vi "Publish Data.vi"(7 "Message Priority (Normal)":T1, 9 "Data":refnum<class "Data.lvclass">, 10 "Actor in":refnum<class "Actor.lvclass">, 11 "Response Msg":refnum<class "Response Msg.lvclass">) -> (0 "error out":errorcluster, 2 "Actor out":refnum<class "Actor.lvclass">)   [LabVIEW 2020, in "Publisher.lvlib" / "Response Msg.lvclass"]
doc: "This Vi handles the publishing of the Data from the Response Msg.\n\nThe default implementation publishes Data if it is non-empty."
uses:
  Response Msg.lvclass
  PPL/HDH.Data.Generic.lvlibp/Data.lvclass
  PPL/HDH.Actor Framework.Core.Actor.lvlibp/1abvi3w/vi.lib/ActorFramework/Actor/Actor.lvclass
  PPL/HDH.Actor Framework.Core.Actor.lvlibp/1abvi3w/vi.lib/ActorFramework/Message Enqueuer/Message Priority.ctl
  Data Msg/Data Msg.lvclass/Data Msg.ctl
  Publisher Messages/Publish Msg/Publish Msg.lvclass/Publish Msg.ctl
  Data Msg/Write Data.vi
  Publisher Messages/Publish Msg/Publish Message.vi
  Data Msg/Data Msg.lvclass
  C:/Current projects/WS/PPL/HDH.Actor Framework.Core.Actor.lvlibp/1abvi3w/vi.lib/ActorFramework/Message/Message.lvclass
  Publisher Messages/Publish Msg/Publish Msg.lvclass
  C:/Current projects/WS/Framework/Framework/Actors/Publisher/Publisher Messages/Publisher Msg/Publisher Msg.lvclass
  Publisher Messages/Publisher Msg/Send To Caller.vi
  PPL/HDH.Actor Framework.Core.Actor.lvlibp/1abvi3w/vi.lib/ActorFramework/Message Enqueuer/Message Enqueuer.lvclass
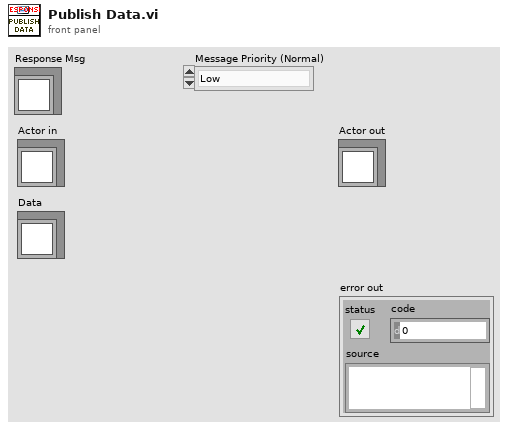
[diagram p1: front panel]
types:
  T1 = typedef "HDH.Actor Framework.Core.Actor.lvlibp/Message Enqueuer.lvclass/Message Priority.ctl" = enum16{"Low", "Normal", "High"}
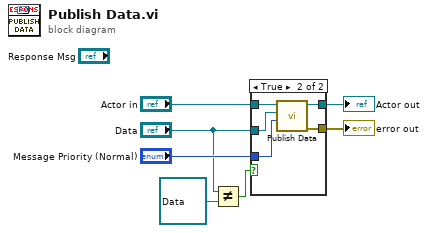
[diagram p0: block diagram]
diagram:
  n1 = Not Equal?(x="Data", y=refnum<class "Data.lvclass"> refnum ("Data")) -> (x != y?=w1:bool)
  n2 = case shown="True" w1 {
    tunnel: [w8 w12] -> w6
    tunnel: "Actor in" -> [w8 w13]
    tunnel: "Data" -> [_ w11]
    tunnel: "Message Priority (Normal)" -> [_ w10]
    tunnel: [_ w9] -> w2
    frame False {
    }
    frame True {
      n3 = call "Publish Data.vi"("Message Priority (Normal)"=w10, "Data to Publish"=w11, "Actor in"=w13) -> ("error out"=w9:errorcluster, "Actor out"=w12:refnum<class "Actor.lvclass">)  [unwired: 6 in, 1 out]
    }
  }
  "Actor out" <- w6
  "error out" <- w2
